vi "e.gate Example - Decode UDBF File.vi"() -> ()   [LabVIEW 2016]
uses:
  e.gate Protocol Type.ctl
  e.gate HighSpeedPort Get File - Read Directory.vi
  e.gate HighSpeedPort Get File - Read FileData.vi
  e.gate Decode UDBF - Stream.vi
panel:
  out "Table":string[][](table)
  in  "DecodeTimeFormat":string
  in  "Index":i32
  in  "Enable Decoding":bool=TRUE
  out "error out":errorcluster
  in  "IP Address":string
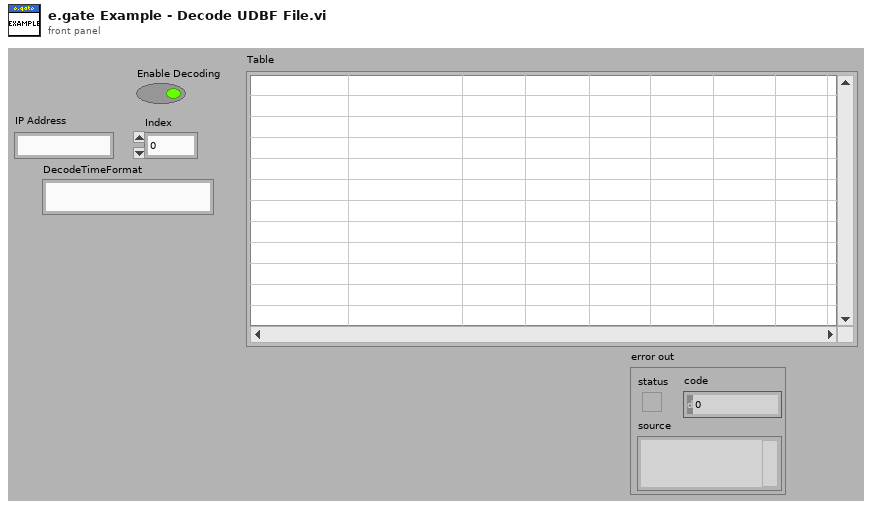
[diagram p1: front panel]
types:
  T1 = enum16{"All Drives", "Flash - Application Files", "Flash - Data", "USB Storage - Data", "Virtual State", "Virtual Circlebuffer", "Virtual Onlinebuffer", "Virtual Archive", "Virtual Logger"}
  T2 = typedef "e.gate Protocol Type.ctl" = enum16{"ASCII", "HighspeedPort Online", "HighspeedPort Buffer", "eGateHighspeedPortDLL "}
  T3 = typedef "e.gate Configuration.ctl" = cluster{"connection ID":refnum<k5>, "IPAddress":string, "BufferIndex":i32, "StateMessage":string, "StateCode":i8, "HeaderSize":i32, "BufferSize":i32, "IsBigEndian":i32, "Version":i32, "ChannelCount":i32, "FrameLength":i32, "StartTime":dbl, "dActTimeToSecondFactor":dbl, "StartTimeToDayFactor":dbl, "BufferFillRate":dbl, "SampleRate":dbl, "ChannelData":T4[], "DecodeTimeFormat":string, "SummaryPath":string, "WithCheckSum":i32, "dActTimeDataType":T5, "MaxWriteCount":i32, "MaxReadCount":i32, "TempOffsetRead":i32, "TempLengthRead":i32, "Protocol":T2, "IsSupported":i32, "InputAccessList":i32[], "OutputAccessList":i32[], "DataSource":enum16{"CircleBuffer", "test.con Logger", "test.con Archive"}, "Modules":T6[], "DLL-Handle":T7}
  T4 = typedef "e.gate Channel Data.ctl" = cluster{"VariableName":string, "DataDirection":string, "DataType":string, "DataTypeIndex":T5, "Precision":i16, "FieldLengtht":i16, "ByteCount":i32, "Format":string, "Unit":string, "InputAccessOffset":i32, "OutputAccessOffset":i16, "InputAccessIndex":i16, "OutputAccessIndex":i16, "VarType":string}
  T5 = typedef "e.gate Data Type.ctl" = enum16{"NO", "BOOL", "SINT8", "USINT8", "SINT16", "USINT16", "SINT32", "USINT32", "FLOAT", "SET8", "SET16", "SET32", "DOUBLE", "SINT64", "USINT64", "SET64"}
  T6 = typedef "e.gate Module  Data.ctl" = cluster{"Type":string, "Location":string, "VariablesCount":i16, "UartIndex":i16, "Address":i16, "SystemOffset":i16}
  T7 = typedef "e.gateHSP_DLLhandle.ctl" = cluster{"clientInstance":i32, "connectionInstance":i32}
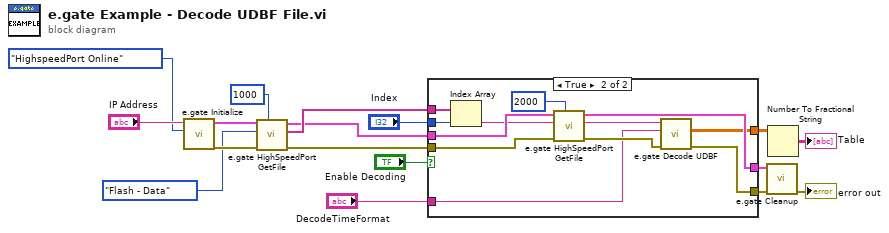
[diagram p0: block diagram]
diagram:
  n1 = call "e.gate Initialize.vi"("Protocol"=e.gate_Protocol_Type."HighspeedPort Online", "IP Address"="IP Address") -> ("error out"=w14:errorcluster, "e.gate Configuration"=w15:T3)  [unwired: 2 in, 6 out]
  n2 = call-poly "e.gate HighSpeedPort GetFile.vi"("Timeout (ms) [1000]"=1000, "error in (no error)"=w14, "Drive Index"=T1."Flash - Data", "Configuration in"=w15) -> ("error out"=w2:errorcluster, "data out"=w3:string[], "Configuration out"=w1:T3)  [unwired: 5 out]
  n3 = case shown="True" "Enable Decoding" {
    tunnel: w1 -> [w19 w30]
    tunnel: [w19 w29] -> w9
    tunnel: w2 -> [w18 w28]
    tunnel: [w18 w31] -> w8
    tunnel: "Index" -> [_ w25]
    tunnel: w3 -> [_ w24]
    tunnel: "DecodeTimeFormat" -> [_ w22]
    tunnel: [_ w21] -> w5
    frame False {
    }
    frame True {
      n4 = Index Array(array=w24, index=w25) -> (element=w23:string)
      n5 = call-poly "e.gate HighSpeedPort GetFile.vi"("Timeout (ms) [1000]"=2000, "error in (no error)"=w28, "File or relative Path"=w23, "Configuration in"=w30) -> ("error out"=w27:errorcluster, "data out (string)"=w26:string, "Configuration out"=w29:T3)  [unwired: 1 in, 4 out]
      n6 = call-poly "e.gate Decode UDBF.vi"("error in (no error)"=w27, "DecodeTimeFormat"=w22, "UDBF Stream"=w26) -> ("error out"=w31:errorcluster, "data array (double)"=w21:dbl[][])  [unwired: 7 out]
    }
  }
  n7 = call "e.gate Cleanup.vi"("error in (no error)"=w8, "e.gate Configuration"=w9) -> ("error out"=→"error out":errorcluster)  [unwired: 9 out]
  n8 = Number To Fractional String(number=w5) -> (F-format string=→"Table":string[][])  [unwired: 3 out]
